vi "potential_compute.vi"(9 "angle":dbl, 10 "distance":cdb, 11 "repulsiveForce":cdb[](array[numeric])) -> (3 "totalForce":cdb[](array[numeric]))   [LabVIEW 2015]
uses:
  <vilib>/imath/engines/lvmath2/RunTimeEngine/ArithmeticOperatorToken/NIMS_ArithmeticOperator_power(S).vi
  <instcachedir>/0/NIMS_ArithmeticOperator_power(S)_DFB67823F1414E5097C86E39787D8CA8.lvgen/NIMS_ArithmeticOperator_power(S)_DFB67823F1414E5097C86E39787D8CA8_009.vi
  <vilib>/imath/engines/lvmath2/RunTimeEngine/BuiltInFunctions/max/1 input/NIMS_max(CV).vi
  <instcachedir>/0/NIMS_max(CV)_A85366AFBDD24459900A7FDE15250013.lvgen/NIMS_max(CV)_A85366AFBDD24459900A7FDE15250013_000.vi
  <vilib>/imathl/engines/lvmath/Functions/Error Handling/Create Error.vi
  <vilib>/imath/engines/lvmath2/RunTimeEngine/ArithmeticOperatorToken/NIMS_ArithmeticOperator_minus.vi
  <instcachedir>/0/NIMS_ArithmeticOperator_minus_8228ED1EA52B4CB8A68367813E4B0C9D.lvgen/NIMS_ArithmeticOperator_minus_8228ED1EA52B4CB8A68367813E4B0C9D_000.vi
  <vilib>/imath/engines/lvmath2/RunTimeEngine/NodeEndStatement/NIMS_NodeEndStatement_Output.vi
  <instcachedir>/0/NIMS_NodeEndStatement_Output_53EC0D466D134D7ABD903AC30B43404B.lvgen/NIMS_NodeEndStatement_Output_53EC0D466D134D7ABD903AC30B43404B_000.vi
  <vilib>/imath/engines/lvmath2/RunTimeEngine/ErrorHandling/NIMS_Finalize Error.vi
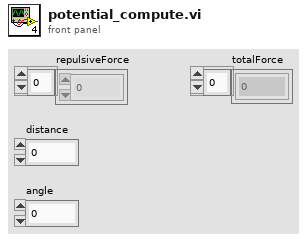
[diagram p1: front panel]
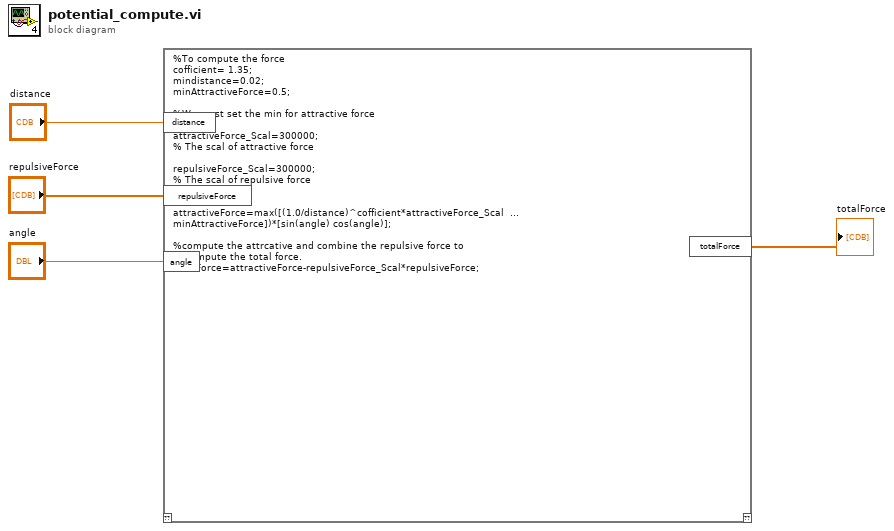
[diagram p0: block diagram]
diagram:
  n1 = mathscript code="%To compute the force \ncofficient= 1.35;      \nmindistance=0.02;\nminAttractiveForce=0.5; \n\n%We must set the min for attractive force             \n\nattractiveForce_Scal=300000; \n% The scal of attractive force\n\nrepulsiveForce_Scal=300000; \n% The scal of repulsive force\n\n\nattractiveForce=max([(1.0/distance)^cofficient*attractiveForce_Scal  ...\nminAttractiveForce])*[sin(angle) cos(angle)];\n\n%compute the attrcative and combine the repulsive force to \n% compute the total force.\ntotalForce=attractiveForce-repulsiveForce_Scal*repulsiveForce;"("distance"="distance", "repulsiveForce"="repulsiveForce", "angle"="angle") -> ("totalForce"=→"totalForce":cdb[])  [unwired: 1 in, 1 out]
